vi "StatusUpdate.vi"(8 "error in (no error)":errorcluster, 9 "Status":string, 11 "Module":refnum<class "ModuleAdmin.lvclass">) -> (0 "error out":errorcluster, 3 "Module":refnum<class "ModuleAdmin.lvclass">)   [LabVIEW 2018, in "DigitizerModule.lvlib"]
uses:
  DigitizerModule.lvlib
  <userlib>/NIST/ModuleAdminLib/ModuleAdmin/ModuleAdmin.lvclass
  clEventType.ctl
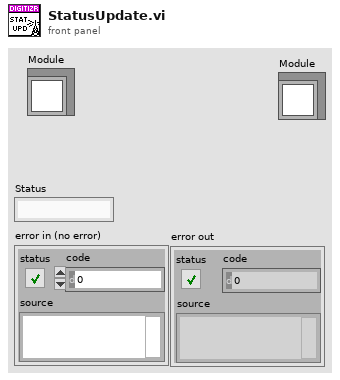
[diagram p1: front panel]
types:
  T1 = typedef "DigitizerModule.lvlib/clEventType.ctl" = cluster{"ModuleID":i32, "Data":variant}
  T2 = typedef "DigitizerModule.lvlib/clBroadcastEvents.ctl" = cluster{"DidInit":refnum<user-event>, "StatusUpdate":refnum<user-event>, "ErrorReport":refnum<user-event>, "DidStop":refnum<user-event>, "PathToINI":refnum<user-event>, "Channels":refnum<user-event>, "Acq":refnum<user-event>, "Trigger":refnum<user-event>, "Waveforms":refnum<user-event>}
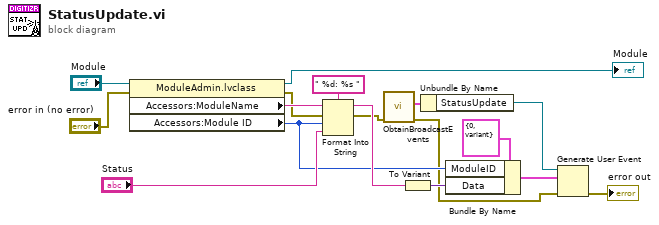
[diagram p0: block diagram]
diagram:
  n1 = property class="ModuleAdmin.lvclass"(reference="Module", error in="error in (no error)") -> (reference out=→"Module":refnum<class "ModuleAdmin.lvclass">, error out=w3:errorcluster, "Accessors:ModuleName"=w9:string, "Accessors:Module ID"=w6:i32)
  n2 = Format Into String(format string=" %d: %s ", initial string=w9, error in=w3, w6, "Status") -> (resulting string=w7:string, error out=w2:errorcluster)
  n3 = call "ObtainBroadcastEvents.vi"("error in (no error)"=w2) -> ("error out"=w1:errorcluster, "clDigitizerBdcstEvents"=w17:T2)  [unwired: 9 in]
  n4 = To Variant(anything=w7) -> (Variant=w14:variant)
  n5 = Unbundle By Name(w17) -> ("StatusUpdate"=w16:refnum<user-event>)
  n6 = Bundle By Name(cluster=T1 {"ModuleID"=0, "Data"=variant} ("clBroadcast"), "ModuleID"=w6, "Data"=w14) -> (w13:T1)
  n7 = Generate User Event(user event=w16, event data cluster=w13, error in=w1) -> (error out=→"error out":errorcluster)  [unwired: 1 in, 1 out]
